vi "Teleop.vi"(10 "Match Info":T1={"Autonomous Elapsed Seconds"=0.0, "TeleOp Elapsed Seconds"=0.0, "Disabled Elapsed Seconds"=0.0, "Visited Autonomous"=FALSE, "Visited TeleOp"=FALSE, "Visited Disabled"=FALSE, "Autonomous Settings"={"Autonomous Style"=enum."Independent", "VI Refnum"=refnum}}, 11 "Call Context":T2) -> ()   [LabVIEW 2017]
doc: "This VI is called for each TeleOp packet received from the DS where the robot is not disabled. It is often used to read from the joysticks and update I/O or to update setpoints for timed control loops. It should complete and return within 20 milliseconds or it may miss DS packets."
uses:
  <vilib>/Rock Robotics/WPI/DriverStation/WPI_DriverStationDerivedRobotMode.ctl
  <vilib>/Rock Robotics/WPI/DriverStation/WPI_DriverStationMatch Info.ctl
  <vilib>/Rock Robotics/WPI/Solenoid/WPI_SolenoidValue.ctl
  <vilib>/Rock Robotics/WPI/Utilities/WPI_GetSetVariantRefNum.vi
  <vilib>/Rock Robotics/Network Tables/NT Write Numeric Array.vi
  <vilib>/Rock Robotics/Network Tables/NT Write Boolean Array.vi
  <vilib>/Rock Robotics/Network Tables/NT Read Boolean.vi
  <vilib>/Rock Robotics/Network Tables/NT Read Number.vi
  <vilib>/Rock Robotics/Network Tables/NT Write Number.vi
  <vilib>/Rock Robotics/WPI/RobotDrive/WPI_RobotDriveArcadeDrive_Standard(NoSaturation).vi
  <vilib>/Rock Robotics/WPI/Solenoid/WPI_SolenoidSetEnum.vi
panel:
  out "Sample Slider 0":dbl(slide) scale=0.0..5.0
  out "Sample Boolean 1":bool
  out "Sample Boolean 0":bool
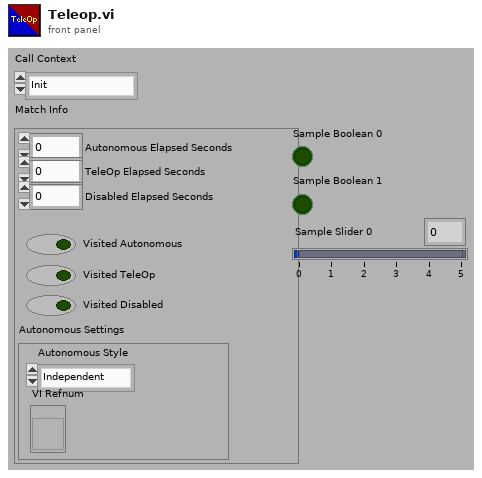
[diagram p1: front panel]
types:
  T1 = typedef "WPI_DriverStationMatch Info.ctl" = cluster{"Autonomous Elapsed Seconds":dbl, "TeleOp Elapsed Seconds":dbl, "Disabled Elapsed Seconds":dbl, "Visited Autonomous":bool, "Visited TeleOp":bool, "Visited Disabled":bool, "Autonomous Settings":cluster{"Autonomous Style":enum16{"Iterative", "Independent"}, "VI Refnum":refnum<vi>}}
  T2 = typedef "WPI_DriverStationDerivedRobotMode.ctl" = enum16{"Init", "Execute", "Stop"}
  T3 = typedef "WPI_SolenoidValue.ctl" = enum16{"Off", "On", "Forward", "Reverse"}
  T4 = typedef "WPI_JoystickDevRef.ctl" = cluster{"Device":T5}
  T5 = typedef "WPI_JoystickDeviceEnum.ctl" = enum16{"USB 0", "USB 1", "USB 2", "USB 3", "USB 4", "USB 5"}
  T6 = cluster{"Axes[0]":dbl, "Axes[1]":dbl, "Axes[2]":dbl, "Axes[3]":dbl, "Axes[4]":dbl, "Axes[5]":dbl, "Axes[6]":dbl, "Axes[7]":dbl, "Axes[8]":dbl}
  T7 = cluster{"Buttons[0]":bool, "Buttons[1]":bool, "Buttons[2]":bool, "Buttons[3]":bool, "Buttons[4]":bool, "Buttons[5]":bool, "Buttons[6]":bool, "Buttons[7]":bool, "Buttons[8]":bool}
  T8 = typedef "WPI_MotorControlDeviceRef.ctl" = cluster{"DeviceStatus":errorcluster, "Type":T9, "PWM":cluster{"PWM Channel":T10, "DeadBand":T11}, "CAN":cluster{"Device Number":u8, "SetOutput VI Ref":variant, "GetOutput VI Ref":variant, "Enable VI Ref":variant, "Disable VI Ref":variant, "Data":variant}, "Invert":bool, "DIO PWM":cluster{"PWM \"Enable\" Channel":T10, "DIOChannel":T12, "PWM Rate":dbl}}
  T9 = typedef "WPI_MotorControlType.ctl" = enum16{"PWM", "CAN", "DIO PWM"}
  T10 = typedef "FPGA_DIOPWMChannel.ctl" = enum8{"PWM 0", "PWM 1", "PWM 2", "PWM 3", "PWM 4", "PWM 5", "PWM 6", "PWM 7", "PWM 8", "PWM 9", "PWM MXP 0", "PWM MXP 1", "PWM MXP 2", "PWM MXP 3", "PWM MXP 4", "PWM MXP 5", "PWM MXP 6", "PWM MXP 7", "PWM MXP 8", "PWM MXP 9", "Invalid"}
  T11 = typedef "WPI_PWMDeadband.ctl" = cluster{"Name":string, "maxPositivePwm":i32, "minPositivePwm":i32, "centerPwm":i32, "maxNegativePwm":i32, "minNegativePwm":i32, "angularRange":u16}
  T12 = typedef "FPGA_DIOChannel.ctl" = enum8{"DIO 0", "DIO 1", "DIO 2", "DIO 3", "DIO 4", "DIO 5", "DIO 6", "DIO 7", "DIO 8", "DIO 9", "DIO MXP 0", "DIO MXP 1", "DIO MXP 2", "DIO MXP 3", "DIO MXP 4", "DIO MXP 5", "DIO MXP 6", "DIO MXP 7", "DIO MXP 8", "DIO MXP 9", "DIO MXP 10", "DIO MXP 11", "DIO MXP 12", "DIO MXP 13", "DIO MXP 14", "DIO MXP 15", "SPI Port CS1", "SPI Port CS2", "SPI Port CS3", "SPI Port MISO", "SPI Port MOSI", "Invalid"}
  T13 = typedef "WPI_RobotDriveDevRef.ctl" = cluster{"DevStatus":errorcluster, "Motors[]":T8[], "Square Inputs":bool, "Max Output":dbl}
  T14 = typedef "WPI_SolenoidDevRef.ctl" = cluster{"DevStatus":errorcluster, "Pneumatics Control Module":u8, "Forward Solenoid Channel":T15, "Reverse Solenoid Channel":T15}
  T15 = typedef "WPI_SolenoidChannel.ctl" = enum8{"Solenoid 0", "Solenoid 1", "Solenoid 2", "Solenoid 3", "Solenoid 4", "Solenoid 5", "Solenoid 6", "Solenoid 7", "Invalid"}
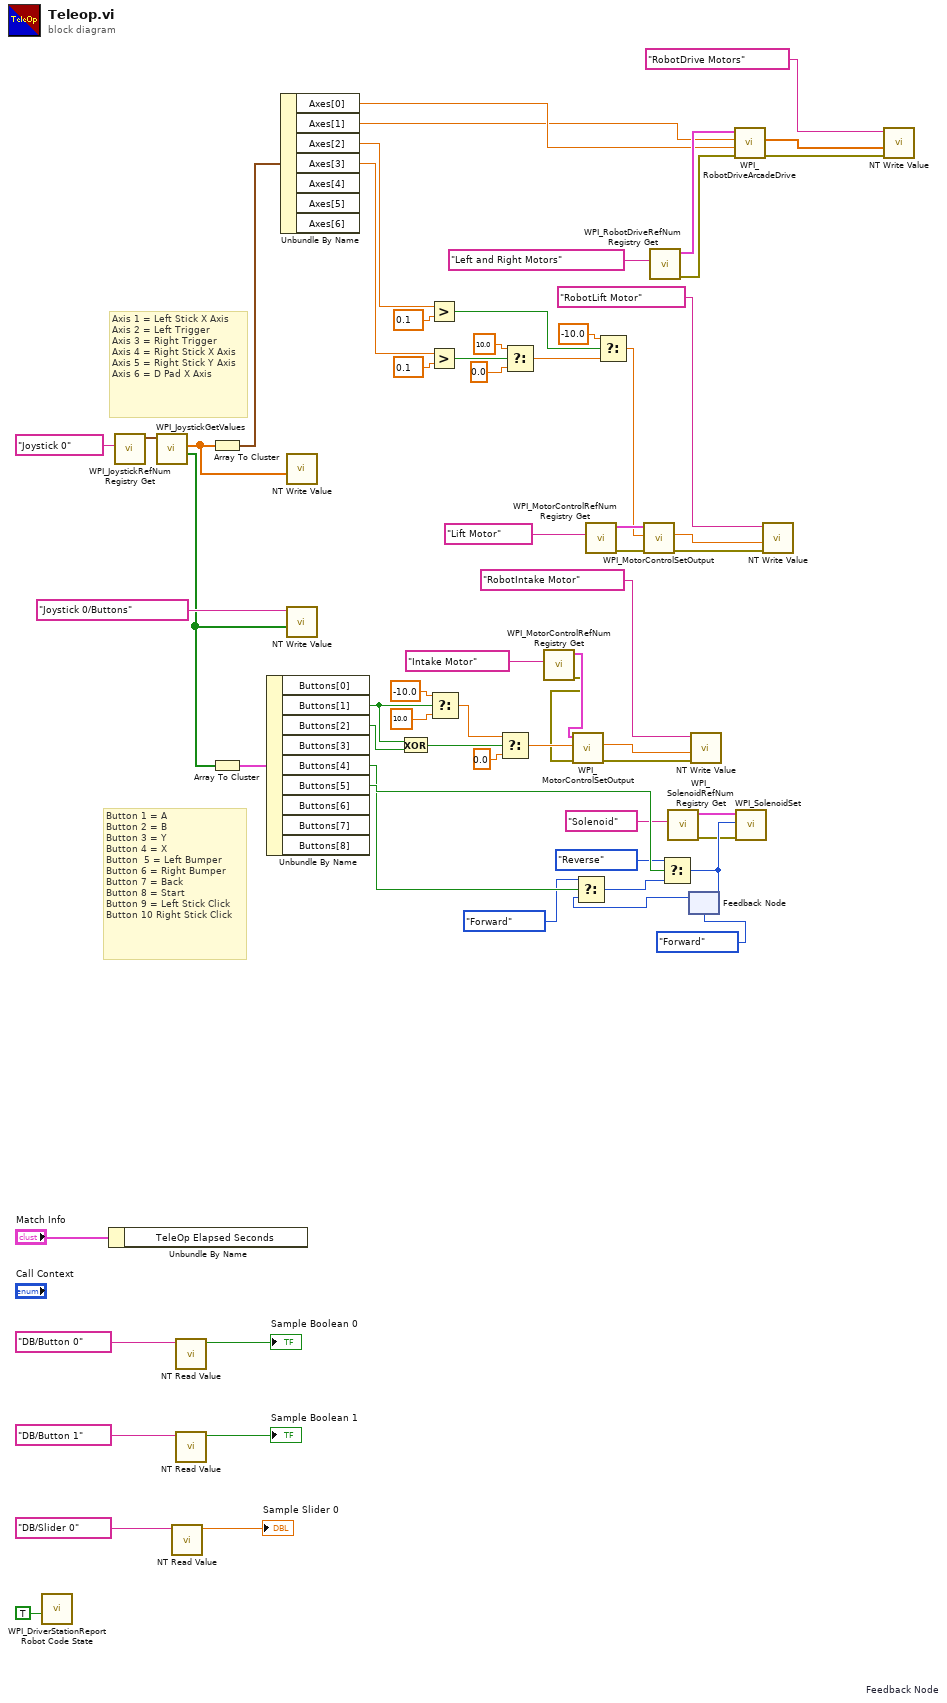
[diagram p0: block diagram]
diagram:
  # "Axis 1 = Left Stick X Axis\nAxis 2 = Left Trigger\nAxis 3 = Right Trigger\nAxis 4 = Right Stick X Axis\nAxis 5 = Right Stick Y Axis\nAxis 6 = D Pad X Axis"
  # "Button 1 = A\nButton 2 = B\nButton 3 = Y\nButton 4 = X\nButton  5 = Left Bumper\nButton 6 = Right Bumper\nButton 7 = Back\nButton 8 = Start\nButton 9 = Left Stick Click\nButton 10 Right Stick Click"
  n1 = call <vilib>:"WPI_DriverStationReport Robot Code State.vi"("TeleOp"=TRUE ("Autonomous")) -> ()  [unwired: 10 in, 1 out]
  n2 = Unbundle By Name("Match Info") -> ()  [unwired: 1 out]
  n3 = call <vilib>:"WPI_JoystickRefNum Registry Get.vi"("refnum name"="Joystick 0") -> ("JoystickDevRef"=w61:T4)  [unwired: 1 in, 9 out]
  n4 = call <vilib>:"WPI_JoystickGetValues.vi"("JoystickDevRef"=w61) -> ("Buttons"=w48:bool[], "Axes"=w50:dbl[])  [unwired: 6 in, 3 out]
  n5 = call-poly <vilib>:"NT Read Value.vi"("Name"="DB/Slider 0" ("refnum name")) -> ("Numeric"=→"Sample Slider 0":dbl)  [unwired: 9 in, 1 out]
  n6 = call-poly <vilib>:"NT Read Value.vi"("Name"="DB/Button 0" ("refnum name")) -> ("Boolean"=→"Sample Boolean 0":bool)  [unwired: 9 in, 1 out]
  n7 = call-poly <vilib>:"NT Read Value.vi"("Name"="DB/Button 1" ("refnum name")) -> ("Boolean"=→"Sample Boolean 1":bool)  [unwired: 9 in, 1 out]
  n8 = Array To Cluster(array=w50) -> (cluster=w49:T6)
  n9 = Array To Cluster(array=w48) -> (cluster=w47:T7)
  n10 = Unbundle By Name(w47) -> ("Buttons[1]"=w43:bool, "Buttons[2]"=w44:bool, "Buttons[4]"=w41:bool, "Buttons[5]"=w42:bool)  [unwired: 5 out]
  n11 = Unbundle By Name(w49) -> ("Axes[0]"=w2:dbl, "Axes[1]"=w1:dbl, "Axes[2]"=w46:dbl, "Axes[3]"=w45:dbl)  [unwired: 3 out]
  n12 = call-poly <vilib>:"NT Write Value.vi"("Numeric Array"=w50) -> ()  [unwired: 10 in, 1 out]
  n13 = call-poly <vilib>:"NT Write Value.vi"("Boolean Array"=w48, "Name"="Joystick 0/Buttons") -> ()  [unwired: 9 in, 1 out]
  n14 = Exclusive Or(1:w44, 2:w43) -> (0:w24:bool)
  n15 = Greater?(x=w46, y=0.1) -> (0:w29:bool)
  n16 = Greater?(x=w45, y=0.1) -> (0:w31:bool)
  n17 = Select(t=-10.0, s=w43, f=10.0) -> (s? t:f=w25:dbl)
  n18 = Select(t=w25, s=w24, f=0.0) -> (s? t:f=w27:dbl)
  n19 = Select(t=10.0, s=w31, f=0.0) -> (s? t:f=w36:dbl)
  n20 = call <vilib>:"WPI_MotorControlRefNum Registry Get.vi"("refnum name"="Intake Motor") -> ("error out"=w4:errorcluster, "MotorControlDevRef"=w22:T8)  [unwired: 9 in]
  n21 = call <vilib>:"WPI_MotorControlSetOutput.vi"("error in (no error)"=w4, "Output"=w27, "MotorControlDevRef"=w22) -> ("error out"=w5:errorcluster, "Motor Output"=w23:dbl)  [unwired: 6 in, 1 out]
  n22 = call <vilib>:"WPI_MotorControlRefNum Registry Get.vi"("refnum name"="Lift Motor") -> ("error out"=w6:errorcluster, "MotorControlDevRef"=w39:T8)  [unwired: 9 in]
  n23 = Select(t=-10.0, s=w29, f=w36) -> (s? t:f=w28:dbl)
  n24 = call <vilib>:"WPI_MotorControlSetOutput.vi"("error in (no error)"=w6, "Output"=w28, "MotorControlDevRef"=w39) -> ("error out"=w7:errorcluster, "Motor Output"=w38:dbl)  [unwired: 6 in, 1 out]
  n25 = call <vilib>:"WPI_RobotDriveRefNum Registry Get.vi"("refnum name"="Left and Right Motors") -> ("error out"=w9:errorcluster, "RobotDriveDevRef"=w63:T13)  [unwired: 1 in, 8 out]
  n26 = call <vilib>:"WPI_SolenoidRefNum Registry Get.vi"("refnum name"="Solenoid") -> ("error out"=w3:errorcluster, "SolenoidDevRef"=w12:T14)  [unwired: 9 in]
  n27 = feedback #1 "Feedback Node"(WPI_SolenoidValue."Forward" ("Value")) -> (w17:T3)
  n28 = Select(t=WPI_SolenoidValue."Forward" ("Value"), s=w41, f=w17) -> (s? t:f=w11:T3)
  n29 = Select(t=WPI_SolenoidValue."Reverse" ("Value"), s=w42, f=w11) -> (s? t:f=w15:T3)
  n30 = feedback-in #1(w15) -> ()
  n31 = call-poly <vilib>:"NT Write Value.vi"("error in"=w5, "Numeric"=w23, "Name"="RobotIntake Motor") -> ()  [unwired: 8 in, 1 out]
  n32 = call-poly <vilib>:"WPI_RobotDriveArcadeDrive.vi"("error in (no error)"=w9, "Y axis value"=w2, "X axis value"=w1, "RobotDriveDevRef"=w63) -> ("error out"=w8:errorcluster, "Motor Values"=w52:dbl[])  [unwired: 5 in, 1 out]
  n33 = call-poly <vilib>:"WPI_SolenoidSet.vi"("error in (no error)"=w3, "Value"=w15, "SolenoidDevRef"=w12) -> ()  [unwired: 7 in, 2 out]
  n34 = call-poly <vilib>:"NT Write Value.vi"("error in"=w7, "Numeric"=w38, "Name"="RobotLift Motor") -> ()  [unwired: 8 in, 1 out]
  n35 = call-poly <vilib>:"NT Write Value.vi"("error in"=w8, "Numeric Array"=w52, "Name"="RobotDrive Motors") -> ()  [unwired: 8 in, 1 out]
